vi "caratterizzazione statica.vi"() -> ()   [LabVIEW 2018]
doc: "This example shows how to configure the oscilloscope to perform an edge-triggered waveform acquisition."
uses:
  <vilib>/Analysis/NI_AALBase.lvlib
  <vilib>/Analysis/NI_AALPro.lvlib
  <vilib>/Analysis/1siggen.llb/Ramp Pattern by Samples.vi
  <vilib>/Analysis/baseanly.llb/Mean (DBL).vi
panel:
  out "max  DNL":dbl=0.25455617495711635
  out "max INL":dbl=0.006364783176684707
  out "INL %":dbl[](array[numeric])=[-0.02405619471115613, 0.06846033804956807, 0.054059831701956974, 0.03454117168943075, -0.03038655836860471, -0.0169696576328108, 0.008050584729997558, 0.03499742026747299, 0.02574456923276381, 0.060912347825317355, 0.034353307326495594, 0.07958518493749565, -0.10774409972043486, -0.021201842595099794, 0.020342897229907505, 0.0016005079430486502, -0.009466821478132525, 0.09116154122292272, -0.01932230466677758, -0.09837062153436701, 0.03364044817915108, -0.011195856420213644, -0.039945564937355474, 0.028477623368902888, 0.029414918163196593, -0.028587533779876415, 0.03593350415287439, 0.03881992615814148, -0.02262514986204033, 0.02136618715120852, 0.040058560181039995, -0.01594928109914272, -0.05257185681596037, -0.03030300195705092, 0.026778203505154082, 0.064704262044265, -0.12952305737290118, 0.041345470255055625, 0.10255372792530139, -0.06324005298613465, 0.020945528396060623, -0.10150639984050625, -0.05126306376498192, -0.004301798179200901, -0.05009188774190607, 0.016201328635920543, 0.030310943352047145, 0.008278932638131297, 0.011989906629121232, 0.005500887190787434, 0.05366077708015016, 0.0719716701814557, -0.008277512747636799, 0.013537732291346796, 0.05896730598852085, -0.05698049429107934, -0.004800590826435734, -0.010604611556285334, -0.05143046497149469, -0.0020644348075213583, -0.024163179746751445, 0.2344907926667456, 0.14697455017375938, 0.20964338602529015, 0.16112184156531656, 0.20423462507496437, 0.18626824583724363, 0.1305633884626625, 0.13010680397133367, 0.18381225454299233, 0.10517732744394762, 0.12992217677058013, 0.17510581294016545, 0.19567783989586932, 0.17998590276065332, 0.11545444986578082, 0.25146759119594675, 0.1749255139529328, 0.12922996766805236, 0.2469189617343613, 0.11945547850968391, 0.19403629983585344, 0.23362332282395698, 0.1956925576555358, 0.11779668279024512, 0.194035727637214, 0.12580094899747457, 0.21720642451959113, 0.2745524121266202, 0.06926517425797794, 0.19953514675634204, 0.05343013134212848, 0.2597150989022119, 0.21261490580646905, 0.16132209405759385, 0.26963134998063487, 0.21786887342412437, 0.09562312790087672, 0.19401450852225913, 0.10571657902932799, 0.17270873155994773, 0.19443092071480667, 0.24458001260962836, 0.1318332034488084, 0.1124323203688547, 0.23550485379434946, 0.2375929283663153, 0.2535110917374496, 0.20460950236283787, 0.2178684745299112, 0.05315797518233562, 0.19460595954160134, 0.3034512313480214, 0.2708214826807394, 0.12574594000636555, 0.14251415541887774, 0.05093588968482587, 0.20449728869005027, 0.1926822373705016, 0.26256355176430085, 0.1411123863773901, 0.19777839159011132, 0.21854781672842588, 0.13600196636201495, 0.13105922904496697, 0.4730276164928865, 0.48395264103777597, 0.4650088701146358, 0.4612302792300106, 0.4427108979968476, 0.41475874913826527, 0.4567820701627306, 0.42666815677927117, 0.4296240398582632, 0.4352469807159263, 0.4348952185112967, 0.4715714849603954, 0.4172577117499153, 0.45106984920335297, 0.39335077022924325, 0.4910664907571427, 0.40855424461403156, 0.46358252844017234, 0.42219567309755557, 0.5061272616143334, 0.4030286187935715, 0.37816665716653164, 0.3520374965638744, 0.4195941282659093, 0.40209211632563824, 0.40889141473324186, 0.3932961304753009, 0.4715090833114835, 0.45913995511626593, 0.3216708713005614, 0.5080044439657493, 0.42130251786092243, 0.4439937536246789, 0.5339617639068427, 0.46177970359606074, 0.431955913497639, 0.3944090090598614, 0.4469254776953338, 0.3251812657824317, 0.4115634438057263, 0.3283808796507927, 0.43996795135533545, 0.40160484810391767, 0.4395084238568267, 0.27704803852776005, 0.4648180517939234, 0.3461999727771157, 0.39272858308450964, 0.4152915571086398, 0.3902766058493558, 0.41615611301747524, 0.48392321491798573, 0.41989782766107037, 0.4661658939641799, 0.3360873621634328, 0.4422271917205249, 0.35287120361413, 0.4864596553968769, 0.4345401946028552, 0.4404514982465365, 0.40099996406206806, 0.41323964167756433, 0.46050567969210243, 0.3250850081180961, 0.29173200579040687, 0.3686345298096912, 0.45417118045506755, 0.47477097934735324, 0.522840701958332, 0.4336171377236045, 0.4631331093354117, 0.49692860692656016, 0.38241450435925395, 0.46634222678171283, 0.38182879987710944, 0.42115342284135643, 0.41682029926610015, 0.44335064761131915, 0.3858182444499899, 0.4345787039660407, 0.3827594146281949, 0.4649047016250239, 0.4882343132461272, 0.4304595205210977, 0.38095777001331044, 0.4465832640416022, 0.42807967259696783, 0.328156912962888, 0.5378848734838563, 0.34536408765170046, 0.47744480430399366, 0.388068448334859, 0.4365205750366294, 0.44042771894135235, 0.4016437108627117, 0.4659221314226296, 0.43530939882665803, 0.4350443527613471, 0.4342764357453131, 0.42212656361326234, 0.47592595132213533, 0.3550740108613398, 0.4073838983181634, 0.3838357698978803, 0.4231175566595142, 0.41826335520964203, 0.36262584640439854, 0.38862935896979195, 0.4000631259067917, 0.40127414514936466, 0.5209281999041453, 0.37808863225516304, 0.331143236282089, 0.4095107639232486, 0.4410859342218857, 0.46127773713094705, 0.4116622392192246, 0.39287821593630257, 0.3538630598555873, 0.44490294875246156, 0.3591077799885698, 0.3665597897571065, 0.6364783176684707]
  out "INL":dbl[](array[numeric])=[-0.0002405619471115613, 0.0006846033804956806, 0.0005405983170195698, 0.0003454117168943075, -0.0003038655836860471, -0.000169696576328108, 8.050584729997559e-05, 0.0003499742026747299, 0.0002574456923276381, 0.0006091234782531735, 0.00034353307326495593, 0.0007958518493749565, -0.0010774409972043486, -0.00021201842595099796, 0.00020342897229907507, 1.60050794304865e-05, -9.466821478132525e-05, 0.0009116154122292272, -0.0001932230466677758, -0.0009837062153436702, 0.0003364044817915108, -0.00011195856420213644, -0.00039945564937355477, 0.0002847762336890289, 0.00029414918163196593, -0.00028587533779876416, 0.00035933504152874395, 0.0003881992615814148, -0.00022625149862040328, 0.00021366187151208518, 0.0004005856018104, -0.0001594928109914272, -0.0005257185681596037, -0.0003030300195705092, 0.0002677820350515408, 0.0006470426204426501, -0.0012952305737290119, 0.00041345470255055625, 0.001025537279253014, -0.0006324005298613465, 0.00020945528396060624, -0.0010150639984050625, -0.0005126306376498193, -4.301798179200902e-05, -0.0005009188774190607, 0.00016201328635920544, 0.00030310943352047145, 8.278932638131298e-05, 0.00011989906629121232, 5.5008871907874336e-05, 0.0005366077708015015, 0.000719716701814557, -8.277512747636798e-05, 0.00013537732291346797, 0.0005896730598852085, -0.0005698049429107934, -4.800590826435734e-05, -0.00010604611556285333, -0.0005143046497149469, -2.0644348075213584e-05, -0.00024163179746751446, 0.002344907926667456, 0.001469745501737594, 0.0020964338602529014, 0.0016112184156531655, 0.0020423462507496437, 0.0018626824583724364, 0.001305633884626625, 0.0013010680397133368, 0.0018381225454299232, 0.0010517732744394761, 0.0012992217677058012, 0.0017510581294016543, 0.001956778398958693, 0.0017998590276065332, 0.0011545444986578082, 0.002514675911959467, 0.0017492551395293279, 0.0012922996766805237, 0.002469189617343613, 0.0011945547850968391, 0.0019403629983585342, 0.0023362332282395697, 0.001956925576555358, 0.0011779668279024511, 0.00194035727637214, 0.0012580094899747457, 0.0021720642451959113, 0.0027455241212662016, 0.0006926517425797794, 0.0019953514675634205, 0.0005343013134212847, 0.002597150989022119, 0.0021261490580646906, 0.0016132209405759384, 0.0026963134998063487, 0.0021786887342412436, 0.0009562312790087672, 0.0019401450852225912, 0.00105716579029328, 0.0017270873155994773, 0.0019443092071480667, 0.0024458001260962837, 0.001318332034488084, 0.001124323203688547, 0.0023550485379434946, 0.002375929283663153, 0.0025351109173744964, 0.0020460950236283787, 0.002178684745299112, 0.0005315797518233562, 0.0019460595954160134, 0.0030345123134802136, 0.0027082148268073943, 0.0012574594000636554, 0.0014251415541887773, 0.0005093588968482586, 0.0020449728869005026, 0.001926822373705016, 0.0026256355176430086, 0.001411123863773901, 0.001977783915901113, 0.0021854781672842587, 0.0013600196636201494, 0.0013105922904496697, 0.004730276164928865, 0.00483952641037776, 0.004650088701146358, 0.004612302792300106, 0.004427108979968476, 0.004147587491382653, 0.004567820701627306, 0.004266681567792712, 0.004296240398582632, 0.004352469807159263, 0.004348952185112967, 0.004715714849603954, 0.004172577117499153, 0.00451069849203353, 0.003933507702292433, 0.004910664907571427, 0.004085542446140316, 0.004635825284401723, 0.004221956730975556, 0.005061272616143334, 0.004030286187935715, 0.0037816665716653166, 0.003520374965638744, 0.004195941282659093, 0.004020921163256383, 0.004088914147332419, 0.003932961304753009, 0.004715090833114835, 0.004591399551162659, 0.0032167087130056137, 0.005080044439657493, 0.004213025178609224, 0.004439937536246789, 0.005339617639068427, 0.004617797035960608, 0.00431955913497639, 0.0039440900905986145, 0.004469254776953338, 0.0032518126578243173, 0.004115634438057263, 0.0032838087965079274, 0.0043996795135533544, 0.004016048481039177, 0.004395084238568267, 0.0027704803852776007, 0.004648180517939234, 0.003461999727771157, 0.003927285830845097, 0.004152915571086398, 0.003902766058493558, 0.004161561130174752, 0.0048392321491798574, 0.004198978276610704, 0.004661658939641799, 0.003360873621634328, 0.004422271917205249, 0.0035287120361413, 0.004864596553968769, 0.004345401946028552, 0.004404514982465365, 0.004009999640620681, 0.0041323964167756435, 0.0046050567969210246, 0.003250850081180961, 0.002917320057904069, 0.003686345298096912, 0.004541711804550676, 0.004747709793473533, 0.005228407019583319, 0.004336171377236045, 0.004631331093354117, 0.004969286069265602, 0.0038241450435925394, 0.004663422267817128, 0.003818287998771094, 0.004211534228413564, 0.004168202992661001, 0.004433506476113192, 0.003858182444499899, 0.004345787039660407, 0.003827594146281949, 0.004649047016250239, 0.004882343132461272, 0.004304595205210977, 0.0038095777001331045, 0.004465832640416022, 0.004280796725969678, 0.0032815691296288804, 0.005378848734838563, 0.003453640876517005, 0.004774448043039937, 0.0038806844833485896, 0.004365205750366294, 0.004404277189413524, 0.004016437108627117, 0.004659221314226296, 0.00435309398826658, 0.004350443527613471, 0.004342764357453131, 0.004221265636132623, 0.0047592595132213535, 0.003550740108613398, 0.004073838983181634, 0.0038383576989788034, 0.0042311755665951425, 0.0041826335520964205, 0.0036262584640439854, 0.0038862935896979193, 0.0040006312590679174, 0.0040127414514936465, 0.0052092819990414525, 0.0037808863225516306, 0.00331143236282089, 0.004095107639232486, 0.004410859342218857, 0.00461277737130947, 0.004116622392192246, 0.003928782159363026, 0.003538630598555873, 0.0044490294875246155, 0.003591077799885698, 0.0036655978975710653, 0.006364783176684707]
  out "LSB":dbl=0.078125
  out "DNL":dbl[](array[numeric])=[-0.114720500623298, 0.017856627871037745, 0.02420313841553252, 0.08051038527196397, -0.016636956912384447, -0.031025100529882367, -0.03341407606646953, 0.011473535283039382, -0.043608045454766396, 0.03293321021853899, -0.05608752823764007, 0.23228831297583383, -0.10731239883541548, -0.05151547738300906, 0.02324056271570498, 0.013723488482264656, -0.1247791697493085, 0.13699996890322835, 0.09801991291581089, -0.16369372644476243, 0.05559701770321226, 0.03564963856125587, -0.08484475349976037, -0.0011622455449241897, 0.07192304040941053, -0.08000608703661101, -0.003579163286531184, 0.07619189426502544, -0.054549257896428574, -0.023178542556991033, 0.06944972318742657, 0.045411993888853884, -0.027613380025047717, -0.0707806947731342, -0.04702831258849756, 0.24084187607728608, -0.21187697425866645, -0.07589823951110475, 0.2055842883301807, -0.10439012091392215, 0.15184039101334293, -0.06230173673365016, -0.05823196932636847, 0.05677971105775441, -0.08220358830850501, -0.017495922247996988, 0.02731969328525565, -0.004601607748827519, 0.00804638410353391, -0.05971826346280977, -0.02270550744561888, 0.0995089868320747, -0.027050903848339657, -0.056332671384495825, 0.14377527234670423, -0.06470308029615808, 0.007196985705013504, 0.050624058234859604, -0.061213877403326934, 0.027402443724645308, -0.3207309257927363, 0.10852014069130292, -0.07770935645589816, 0.06016671513036727, -0.05345985155196331, 0.022278310254773715, 0.06907402314448063, 0.0005661647692477345, -0.06659475870885671, 0.09750730960281544, -0.030683613165024326, -0.05602770885028576, -0.025509313425072833, 0.019458002047667834, 0.0800190015896419, -0.16865629524940573, 0.09491217578133729, 0.05666247739325172, -0.14593435264222307, 0.15805471919859998, -0.0924802184444502, -0.04908790850524838, 0.04703414880884225, 0.09659088483296045, -0.09453641561024143, 0.08461112551327687, -0.11334278964742453, -0.071109024632716, 0.25455617495711635, -0.1615347658979715, 0.18117021911362485, -0.2557933597745034, 0.058404239438721105, 0.06360308656860525, -0.13430347734457088, 0.06418547093007305, 0.15158472444882704, -0.12200531197051419, 0.1094894325712346, -0.08307026913796847, -0.026935514552025096, -0.0621848739495789, 0.13980604335941677, 0.024057095019142594, -0.15260994144761356, -0.0025892124692376227, -0.019738522580206565, 0.060637970824518564, -0.016441125487170895, 0.20424101919099372, -0.17539550060548947, -0.13496813703996083, 0.0404608883474296, 0.17989367291622357, -0.020792587111515104, 0.11355704951022431, -0.19041613476647826, 0.014650663636240324, -0.08665282984831109, 0.15059944507976936, -0.07026584646377429, -0.025754087171510065, 0.10235685445434957, 0.006128994273139554, -0.4240408004354202, -0.013547030435663032, 0.023490275944693904, 0.004685452696935144, 0.022964032729122154, 0.03466066458464212, -0.05210891807033704, 0.037341252595489746, -0.003665295017950143, -0.006972446663502297, 0.00043618513374070743, -0.04547857039688239, 0.06734907878099534, -0.04192705044226273, 0.07157165792789613, -0.12116749345459539, 0.10231518521745783, -0.06823507194441447, 0.0513197006248447, -0.10407516976080444, 0.12784231709774474, 0.030828832417529383, 0.03240015914729497, -0.0837702233105233, 0.021702494805936112, -0.008431130025428502, 0.019338152479846826, -0.09698406151686641, 0.015337718962069858, 0.1704616639314736, -0.231053630104833, 0.10751038836998532, -0.028137132347058013, -0.11156033274988317, 0.08950575478536962, 0.03698149972204305, 0.046558161502844086, -0.06512042110798574, 0.15096282277199863, -0.10711390074888527, 0.10314637955211765, -0.13836796891363293, 0.04757024803175795, -0.04700043393360716, 0.2014508778080426, -0.2328348164500426, 0.1470864179808416, -0.05769547678116851, -0.027978087789921346, 0.03101853956151217, -0.03209058888846812, -0.084031206356633, 0.07939148019857498, -0.0573724022158558, 0.16129737943292638, -0.13161338865079414, 0.11080142525192968, -0.16564968021060622, 0.06438013138458701, -0.007330016518164939, 0.04891990238874087, -0.015177200243215339, -0.05860988713802726, 0.1679216327517679, 0.041357722886334616, -0.09535912978391252, -0.10606544680026672, -0.025543750626434304, -0.0596064560376135, 0.11063721965106196, -0.03659980479864089, -0.04190641701302411, 0.14199748718345973, -0.10407037580384895, 0.10479664936170821, -0.04876253247566638, 0.005373073233317882, -0.032897631948071646, 0.07134017992004829, -0.060462969799903024, 0.06425591877892885, -0.10186015587606789, -0.02892871841016813, 0.07164074297903653, 0.06138217062965623, -0.08137561259508175, 0.022944453391346542, 0.12390422194625898, -0.26006267104600056, 0.2387257744318731, -0.1637800886488435, 0.110826681401727, -0.06008063711019531, -0.004844858441856559, 0.04809217001751449, -0.07970524149429821, 0.037959788419004784, 0.00032865712098555376, 0.0009522170998820911, 0.015065841443743011, -0.06671124075900252, 0.14985640617138643, -0.06486426044646124, 0.029199679241150987, -0.0487094155844261, 0.00601920979784154, 0.06899051091850197, -0.032244355581087805, -0.014177871001879793, -0.0015016638607903588, -0.1483710278959279, 0.17712106388473786, 0.05821229100661185, -0.09717573427503794, -0.03915321117030999, -0.025037835607236048, 0.06152321741053583, 0.02329218887082334, 0.048378793540086916, -0.11288946223212407, 0.10638600926722575, -0.009240492112985521, -0.3346989746100917]
  in  "Tab Control":T1(tab)=enum."CONFRONTO IDEALE E REALE"
  out "confonto":waveform(dbl)[](graph)=[{"t0"=timestamp(0 s since 1904-01-01), "dt"=0.004968040310037549, "Y"=array[248 elements]}, {"t0"=timestamp(0 s since 1904-01-01), "dt"=0.004968040310037549, "Y"=array[248 elements]}]
  out "caratteristica statica":cluster{dbl[], dbl[]}(graph)
  out "confronto_rette":waveform(dbl)[](graph)=[{"t0"=timestamp(0 s since 1904-01-01), "dt"=0.004968040310037549, "Y"=array[248 elements]}, {"t0"=timestamp(0 s since 1904-01-01), "dt"=0.004968040310037549, "Y"=array[248 elements]}]
  out "errore di guadagno":dbl=-0.03778591631762984
  out "errore di offset":dbl=-0.0867022391606219
  out "indice di fine":i32[](array[numeric])=[14456, 16723, 18456, 21505, 23709, 26413, 29108, 31158, 33625, 36266, 38593, 40967, 43393, 45899, 48260, 50985, 53393, 55786, 58394, 61024, 63323, 65806, 68077, 70558, 73011, 75148, 77531, 80438, 83009, 85630, 87816, 89884, 92915, 95362, 97565, 100055, 102725, 105116, 107615, 109890, 112715, 114748, 117411, 119927, 122388, 124611, 127009, 129720, 132220, 134440, 137028, 139689, 142241, 144479, 147120, 149302, 151791, 154288, 156401, 158906, 161200, 161840, 163991, 166805, 168779, 171154, 173963, 176799, 178820, 181316, 183821, 186240, 188493, 190897, 193657, 195968, 198386, 200815, 203476, 205711, 208132, 210856, 213165, 215518, 218224, 220352, 223130, 225234, 227710, 230461, 232827, 235213, 237556, 240076, 242612, 245335, 247884, 249961, 252449, 255007, 257485, 260368, 262124, 264905, 267237, 269451, 272112, 274533, 276764, 279531, 281913, 284275, 286601, 289404, 291680, 294136, 296699, 299289, 301701, 304247, 306668, 309055, 311414, 313809, 316282, 318363, 320936, 323678, 325761, 328350, 330813, 333525, 335679, 338193, 340678, 343038, 345661, 347935, 350198, 352729, 355358, 357454, 360316, 362728, 364986, 367659, 369996, 372569, 374882, 377422, 379681, 382098, 384776, 386954, 389560, 392053, 394753, 397195, 399599, 402323, 404450, 406924, 409239, 411743, 414037, 416556, 419129, 421576, 424003, 426770, 428845, 431509, 433963, 436150, 438972, 441177, 443554, 446420, 448927, 451100, 453904, 456074, 458409, 460997, 463092, 465352, 467869, 470586, 472925, 474843, 477222, 479813, 482368, 484728, 487359, 489650, 492193, 494678, 497046, 499683, 502458, 504340, 506860, 509357, 512055, 514236, 517014, 519521, 521613, 524185, 526630, 529244, 531831, 533968, 536546, 538865, 541776, 543881, 546333, 548925, 551386, 554006, 556481, 558698, 561061, 563619, 566039, 568728, 571076, 573756, 576131, 578465, 580633, 583168, 585776, 588224, 590660, 593170, 596000, 598189, 600599, 602951, 605989, 607859, 610435, 612874, 615271, 616036]
  out "min value":dbl=-9.765625
  out "max value":dbl=9.6875
  out "numeri di bit eq":dbl=8.0
  out "Mediane\n delle transizioni":dbl[](array[numeric])=[-9.711754383605852, -9.628450693829347, -9.563160577563249, -9.482094657483247, -9.402734254100897, -9.318823887343532, -9.240546693360889, -9.173558042212518, -9.086142774343122, -8.999841370558375, -8.933272006793093, -8.856738023732786, -8.773977577473183, -8.697079406873614, -8.61836308611707, -8.537818585337915, -8.45963081566549, -8.380008308714919, -8.305852108986114, -8.226776401564537, -8.147385386819485, -8.063110453034081, -7.992749471086037, -7.918102548036758, -7.8318115234375, -7.758912816811036, -7.6826498035363455, -7.605517818132168, -7.524312187775492, -7.438687001182383, -7.370851277101277, -7.2942079835606854, -7.208347315436241, -7.13753003203417, -7.0553024933288855, -6.977843198016734, -6.8980551010244735, -6.818803543613707, -6.747076277068295, -6.668486563773111, -6.580164210074413, -6.518291975881262, -6.435745709714951, -6.351214960390006, -6.269655577447711, -6.205167767732963, -6.117637662639405, -6.041772527100271, -5.962948616315941, -5.889512310606061, -5.8112699370793095, -5.726219533922463, -5.643830796497081, -5.5773093250070165, -5.495097268790165, -5.415857919254658, -5.332570329087049, -5.255821078431373, -5.181534090909091, -5.102868210306407, -5.019800275482094, -4.966740262681159, -4.88468137254902, -4.793696609717031, -4.726530136702569, -4.655189479638009, -4.563558467741935, -4.4846746333897345, -4.408865770210057, -4.332170514319111, -4.262139545223577, -4.178438065781533, -4.108913745387454, -4.017409500339904, -3.9443576860401954, -3.869053002894356, -3.7851304188096986, -3.715886377613776, -3.634807378266033, -3.5635558684054534, -3.4804461994868507, -3.3906963005215123, -3.317048373287671, -3.237247816139767, -3.1634347960444993, -3.0865077554744524, -3.007653617083091, -2.9284452296819787, -2.8515897212543555, -2.770127118644068, -2.697134067357513, -2.619495476366322, -2.5488352479941647, -2.4585282397782398, -2.393628003003003, -2.301866460637606, -2.2168218510230178, -2.1481579830053668, -2.0776494060876023, -1.9934338521400778, -1.9142027099784638, -1.8290969681129117, -1.7661413257277734, -1.6785218598195697, -1.6078115638106651, -1.5233654289667897, -1.4471704345273046, -1.3757402368758003, -1.2886949315654406, -1.2061106687898089, -1.133898384673178, -1.0544518288084463, -0.9794178598342125, -0.8953067200986436, -0.8196829432079816, -0.7485795454545454, -0.6641673657718121, -0.5897458217270195, -0.5060948581560284, -0.42627245508982037, -0.3540540072102052, -0.2712673611111111, -0.1934148264984227, -0.12478081162324649, -0.04931294326241135, 0.01962819778541428, 0.09187700029095142, 0.17405523255813954, 0.2466143428747307, 0.3293353873239437, 0.409167921686747, 0.49038392343120324, 0.5589087511325883, 0.6450269033087054, 0.7237224430113978, 0.7991752001847859, 0.8738205946239479, 0.9510988609813084, 1.0331075174825175, 1.1025232812927965, 1.193955866727383, 1.2645524222381124, 1.3461640869071287, 1.4225535558146314, 1.4956722474905897, 1.5865265376984128, 1.6529498922413792, 1.7277175350436393, 1.8039060323209808, 1.8990197224820704, 1.9655420676582094, 2.050463237788331, 2.117670203790239, 2.208102154046997, 2.289998811033608, 2.359254360880755, 2.4440541714947854, 2.518349723090031, 2.591874651907547, 2.674368564993565, 2.745297585626053, 2.8192620103229222, 2.902835700330628, 2.9789595170454546, 3.05321250721709, 3.12722255770263, 3.219967995759948, 3.2934160656461584, 3.3678232758620688, 3.4548046980774436, 3.516169717082328, 3.6074509410563174, 3.685823516889015, 3.7612781268264173, 3.839204616637434, 3.9180570610096006, 3.9940007831145583, 4.08481835399449, 4.160177342062635, 4.234902426160337, 4.321937769010043, 4.384071021928592, 4.468474860982391, 4.561700386789646, 4.618910424305919, 4.692457507082153, 4.771928792361485, 4.861704465541491, 4.941709844559585, 5.014073149951314, 5.095332829925651, 5.174446749654218, 5.246905979918658, 5.329749888259833, 5.40919678147939, 5.48263143776824, 5.5652769866135, 5.638174862448418, 5.716356402528668, 5.799642559689062, 5.8805637406947895, 5.946947782920275, 6.02677319876647, 6.109089921807124, 6.182066077760892, 6.266436002764128, 6.347696603822314, 6.420555134041477, 6.502976190476191, 6.584933483935743, 6.654728084415584, 6.731294775197629, 6.808154273297924, 6.8862526633522725, 6.971515326778484, 7.045321377840909, 7.131132309217047, 7.201062620556627, 7.2745652887139105, 7.362013813467282, 7.432948435972629, 7.525845390309556, 7.591424546713674, 7.675149150049036, 7.750260569046226, 7.825229960578187, 7.901683293937708, 7.986540421195652, 8.056343454879329, 8.140026325805634, 8.221902105484052, 8.29412798272079, 8.376196997162673, 8.455096316680779, 8.523932963588136, 8.610032306846302, 8.686717692828147, 8.766010641985579, 8.851975565582105, 8.915021315658452, 8.999592391304347, 9.078675560570764, 9.160938219052001, 9.22901774003148, 9.310064409632314, 9.389618288590604, 9.47034502423724, 9.521046789617486]
  out "indice di inizio":i32[](array[numeric])=[9808, 13336, 15452, 17476, 20478, 22818, 25237, 27723, 30390, 32917, 35060, 37554, 40037, 42291, 44997, 47493, 49997, 52401, 54577, 57189, 59833, 62197, 64532, 66967, 69811, 72031, 74477, 76776, 79606, 82247, 84449, 87025, 89190, 91616, 94567, 96828, 99211, 101906, 104013, 106699, 109221, 111514, 113973, 116645, 119089, 121016, 123781, 126030, 128751, 131140, 133611, 136181, 138644, 140916, 143541, 146082, 148494, 150616, 153101, 155316, 157933, 160184, 162716, 164932, 167572, 170049, 172413, 175026, 177249, 179605, 181853, 184583, 187138, 189426, 191816, 194586, 197025, 199189, 201792, 204024, 206573, 209322, 211705, 214316, 216606, 218982, 221409, 224102, 226275, 228986, 231476, 233859, 236185, 238633, 240947, 243798, 246320, 248843, 251102, 253722, 256092, 258455, 260853, 263464, 265568, 268367, 270409, 272971, 275595, 277961, 280582, 282949, 285274, 287782, 290377, 292541, 295209, 297494, 300291, 302577, 304865, 307579, 309829, 312312, 314449, 315744, 317499, 320023, 322512, 324800, 327493, 330051, 332368, 335080, 337344, 339791, 341978, 344511, 347195, 349078, 352064, 354657, 356795, 359297, 361798, 364635, 366516, 368788, 371293, 374215, 376252, 379150, 380924, 384273, 386406, 388556, 391301, 393674, 396008, 398438, 400888, 403146, 405912, 408223, 410573, 412830, 416063, 418179, 420378, 423077, 425116, 428082, 430440, 432728, 434981, 437948, 440202, 442790, 445223, 447782, 450419, 452517, 455172, 457636, 459274, 461822, 464151, 467031, 469644, 471762, 473994, 476198, 478434, 481372, 483817, 486155, 488682, 491043, 493645, 496081, 498428, 500991, 503293, 505904, 508107, 510980, 513142, 515567, 518442, 520699, 522780, 525196, 527689, 530448, 533088, 535345, 537740, 540252, 542523, 545242, 547294, 550291, 552510, 555639, 557643, 559814, 562443, 565048, 567264, 569815, 572557, 574819, 577461, 579625, 581629, 584587, 586965, 589564, 592066, 594172, 597149, 599517, 601643, 604047, 606573, 609149, 611764, 614206]
  out "RAMPA":dbl[](graph)
  in  "length":i32=1400000
  in  "Vertical Coupling (0: A1M)":u16(ring)=2 items=["A1M", "A50", "D1M", "D50", "Ground"]
  in  "Probe Attenuation (1X)":dbl=1.0
  in  "Vertical Range (1 V)":dbl=2.0
  in  "Trigger Level (0.0 V)":dbl
  in  "Timebase (0.0005 s)":dbl=0.2
  in  "Source (1: Channel 1)":u16(ring)=1 items=["Channel 1"=1, "Channel 2"=2, "Channel 3"=3, "Channel 4"=4]
  in  "VISA resource name":refnum<visa-resource-name>="USB0::0xF4EC::0xEE38::SDSMMEBX3R2562::INSTR"
  # "PARAMETRI DELL'ADC"
  # "CARATTERIZZAZIONE STATICA"
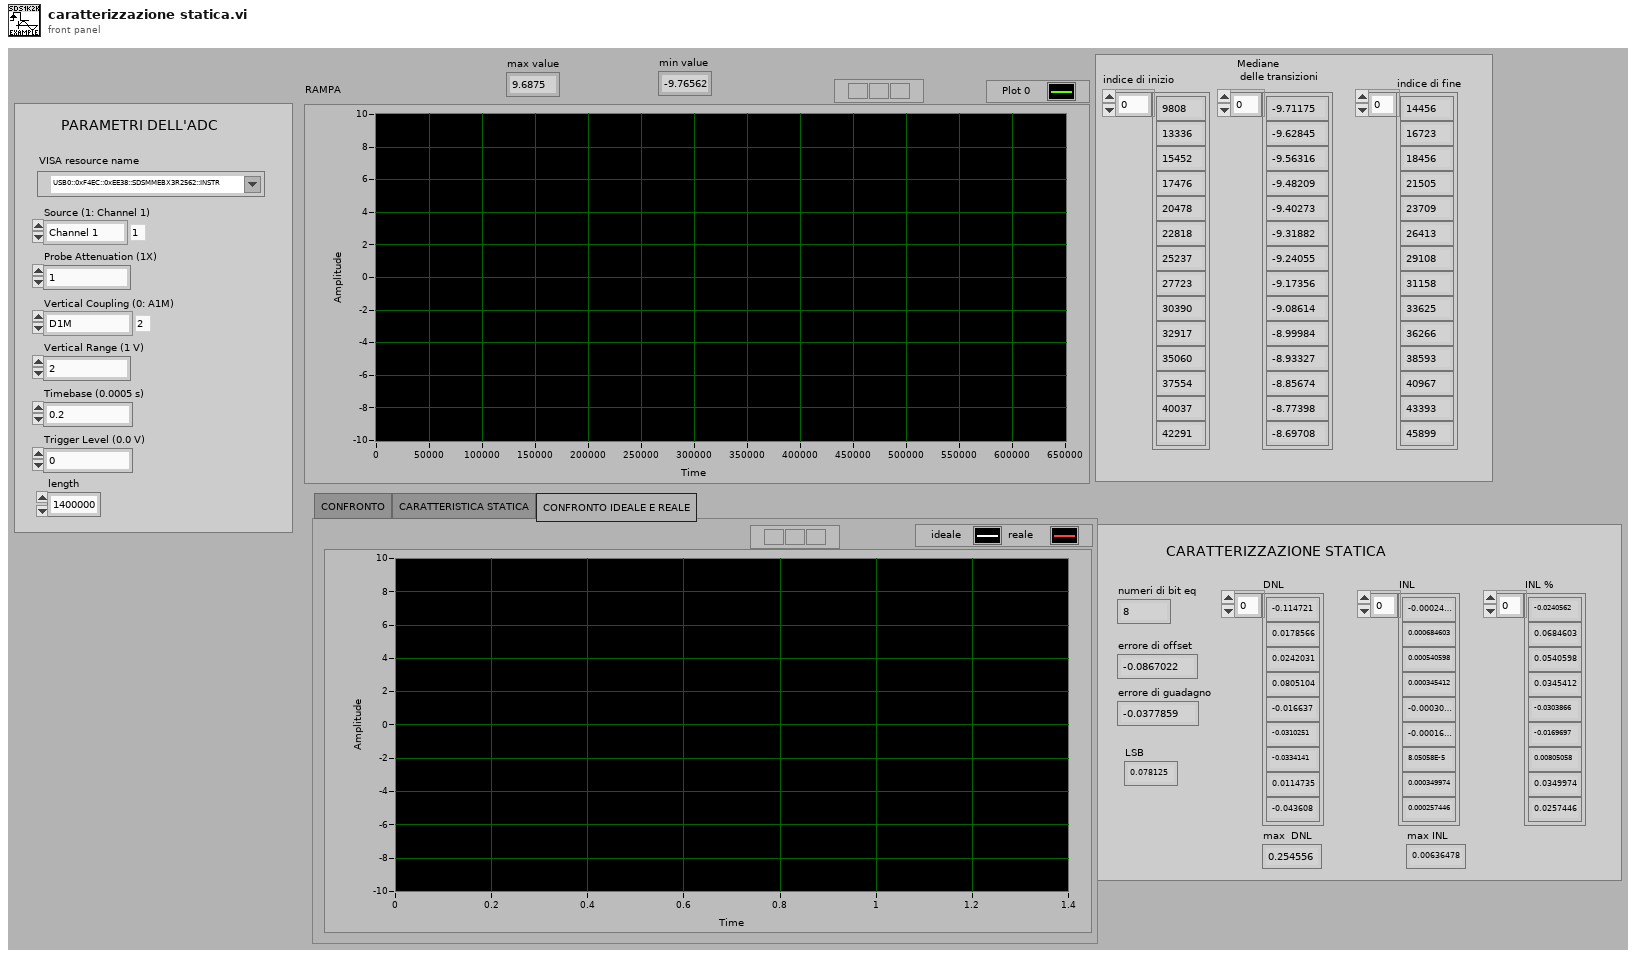
[diagram p1: front panel]
types:
  T1 = enum32{"CONFRONTO", "CARATTERISTICA STATICA", "CONFRONTO IDEALE E REALE"}
  T2 = cluster{"Best Linear Fit":dbl[], "Ramp Pattern":dbl[]}
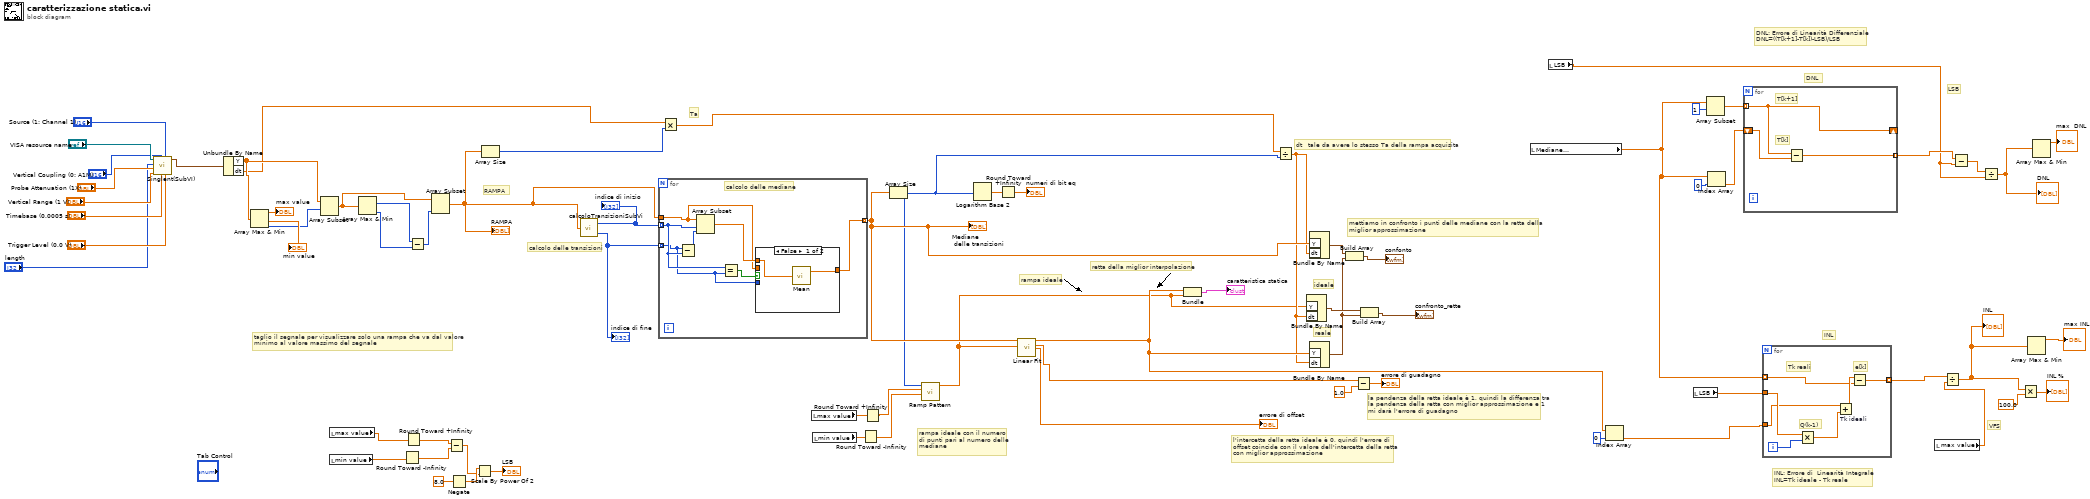
[diagram p0: block diagram]
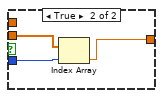
[diagram p2: hidden frame]
diagram:
  # "reale"
  # "ideale"
  # "INL: Errore di  Linearità Integrale\nINL=Tk ideale - Tk reale"
  # "VFS"
  # "INL"
  # "DNL: Errore di Linearità Differenziale\nDNL=((T[k+1]-T[k])-LSB)/LSB"
  # "LSB"
  # "DNL"
  # "rampa ideale con il numero\ndi punti pari al numero delle\nmediane"
  # "mettiamo in confronto i punti delle mediane con la retta della\nmiglior approssimazione"
  # "la pendenza della retta ideale è 1, quindi la differenza tra\nla pendenza della retta con miglior approssimazione e 1 \nmi darà l'errore di guadagno"
  # "l'intercetta della retta ideale è 0, quindi l'errore di \noffset coincide con il valore dell'intercetta della retta\ncon miglior approssimazione"
  # "rampa ideale"
  # "retta della miglior interpolazione"
  # "RAMPA"
  # "taglio il segnale per visualizzare solo una rampa che va dal valore\nminimo al valore massimo del segnale"
  # "calcolo delle transizioni"
  # "dt   tale da avere lo stesso Ta della rampa acquisita"
  # "Ta"
  n1 = call "Singlent(SubVI).vi"("Trigger Level (0.0 V)"="Trigger Level (0.0 V)", "Source (1: Channel 1)"="Source (1: Channel 1)", "Timebase (0.0005 s)"="Timebase (0.0005 s)", "Vertical Coupling (0: A1M)"="Vertical Coupling (0: A1M)", "Vertical Range (1 V)"="Vertical Range (1 V)", "Probe Attenuation (1X)"="Probe Attenuation (1X)", "length"="length", "VISA Refnum in"="VISA resource name") -> ("Waveform Graph"=w5:waveform(dbl))  [unwired: 3 in]
  n2 = Unbundle By Name(w5) -> ("Y"=w60:dbl[], "dt"=w47:dbl)
  n3 = Array Max & Min(array=w60) -> (max value=→"max value":dbl, min value=→"min value":dbl, min index (indices)=w55:i32)  [unwired: 1 out]
  n4 = Array Subset(array=w60, index=w55) -> (w51:dbl[])  [unwired: 1 in]
  n5 = local read "max value"() -> (w13:dbl)
  n6 = local read "min value"() -> (w12:dbl)
  n7 = Array Max & Min(array=w51) -> (max index (indices)=w52:i32, min index (indices)=w53:i32)  [unwired: 2 out]
  n8 = Round Toward -Infinity(1:w12) -> (0:w14:dbl)
  n9 = Round Toward +Infinity(x=w13) -> (ceil(x): smallest int >= x=w15:dbl)
  n10 = Subtract(x=w52, y=w53) -> (x-y=w54:i32)
  n11 = Array Subset(array=w51, length=w54) -> (w48:dbl[])  [unwired: 1 in]
  "RAMPA" <- w48
  n12 = Subtract(x=w15, y=w14) -> (x-y=w30:dbl)
  n13 = Negate(x=8.0) -> (-x=w31:dbl)
  n14 = Scale By Power Of 2(n=w31, x=w30) -> (x*2^n=→"LSB":dbl)
  n15 = Array Size(array=w48) -> (size(s)=w7:i32)
  n16 = call "calcoloTransizioniSubVi.vi"("Array"=w48) -> ("indice di inizio"=w57:i32[], "indice di fine"=w56:i32[])
  "indice di inizio" <- w57
  "indice di fine" <- w56
  n17 = for {
    tunnel: w48 -> [w74]
    tunnel: w57 -> [w73] mode=indexing
    tunnel: w56 -> [w72] mode=indexing
    tunnel: [w75] -> w45 mode=indexing
    # "calcolo delle mediane"
    n18 = Subtract(x=w72, y=w73) -> (x-y=w78:i32)
    n19 = Array Subset(array=w74, index=w73, length=w78) -> (w76:dbl[])
    n20 = Equal?(x=w73, y=w72) -> (x = y?=w77:bool)
    n21 = case shown="False" w77 {
      tunnel: w76 -> [w80 _]
      tunnel: [w79 w83] -> w75
      tunnel: w74 -> [_ w82]
      tunnel: w72 -> [_ w81]
      frame False {
        n22 = call-poly <vilib>:"Mean.vi"("X"=w80) -> ("mean"=w79:dbl)  [unwired: 1 out]
      }
      frame True {
        n23 = Index Array(array=w82, index=w81) -> (element=w83:dbl)
      }
    }
  }
  "Mediane\n delle transizioni" <- w45
  n24 = Multiply(x=w47, y=w7) -> (x*y=w46:dbl)
  n25 = local read "max value"() -> (w43:dbl)
  n26 = local read "min value"() -> (w42:dbl)
  n27 = Round Toward -Infinity(1:w42) -> (0:w16:dbl)
  n28 = Round Toward +Infinity(x=w43) -> (ceil(x): smallest int >= x=w17:dbl)
  n29 = Array Size(array=w45) -> (size(s)=w44:i32)
  n30 = call-poly <vilib>:"Ramp Pattern.vi"("start"=w16, "end"=w17, "samples"=w44) -> ("Ramp Pattern"=w6:dbl[])  [unwired: 7 in, 1 out]
  n31 = Logarithm Base 2(1:w44) -> (0:w63:dbl)
  n32 = Round Toward +Infinity(x=w63) -> (ceil(x): smallest int >= x=→"numeri di bit eq":dbl)
  n33 = call <vilib>:"Linear Fit.vi"("Y"=w45, "X"=w6) -> ("Best Linear Fit"=w19:dbl[], "slope"=w40:dbl, "intercept"=→"errore di offset":dbl)  [unwired: 9 in, 2 out]
  n34 = Bundle("Best Linear Fit"=w19, "Ramp Pattern"=w6) -> (→"caratteristica statica":T2)  [unwired: 1 in]
  n35 = Divide(x=w46, y=w44) -> (x/y=w11:dbl)
  n36 = Bundle By Name("Y"=w6, "dt"=w11) -> (w10:waveform(dbl))  [unwired: 1 in]
  n37 = Bundle By Name("Y"=w45, "dt"=w11) -> (w50:waveform(dbl))  [unwired: 1 in]
  n38 = Bundle By Name("Y"=w19, "dt"=w11) -> (w9:waveform(dbl))  [unwired: 1 in]
  n39 = Build Array(w50, w9) -> (→"confonto":waveform(dbl)[])
  n40 = Subtract(x=w40, y=1.0) -> (x-y=→"errore di guadagno":dbl)
  n41 = Build Array(w10, w9) -> (→"confronto_rette":waveform(dbl)[])
  n42 = local read "Mediane\n delle transizioni"() -> (w21:dbl[])
  n43 = local read "LSB"() -> (w27:dbl)
  n44 = Index Array(array=w19, index=0) -> (element=w18:dbl)
  n45 = local read "LSB"() -> (w22:dbl)
  n46 = Array Subset(array=w21, index=1) -> (w35:dbl[])  [unwired: 1 in]
  n47 = Index Array(array=w21, index=0) -> (element=w33:dbl)
  n48 = for {
    tunnel: w35 -> [w86] mode=indexing
    shift-right: [w86] -> _
    shift-left: w33 -> [w85]
    tunnel: [w84] -> w32 mode=indexing
    # "T[k]"
    # "T[k+1]"
    n49 = Subtract(x=w86, y=w85) -> (x-y=w84:dbl)
  }
  n50 = for {
    tunnel: w18 -> [w90]
    tunnel: w21 -> [w87] mode=indexing
    tunnel: w22 -> [w92]
    tunnel: [w89] -> w23 mode=indexing
    i -> [w93]
    # "Tk reali"
    # "e[k]"
    # "Q(k-1)"
    n51 = Multiply(x=w92, y=w93) -> (x*y=w91:dbl)
    n52 = Add "Tk ideali"(x=w90, y=w91) -> (x+y=w88:dbl)
    n53 = Subtract(x=w88, y=w87) -> (x-y=w89:dbl)
  }
  n54 = local read "max value"() -> (w25:dbl)
  n55 = Divide(x=w23, y=w25) -> (x/y=w3:dbl[])
  "INL" <- w3
  n56 = Subtract(x=w32, y=w27) -> (x-y=w34:dbl[])
  n57 = Divide(x=w34, y=w27) -> (x/y=w4:dbl[])
  "DNL" <- w4
  n58 = Multiply(x=w3, y=100.0) -> (x*y=→"INL %":dbl[])
  n59 = Array Max & Min(array=w3) -> (max value=→"max INL":dbl)  [unwired: 3 out]
  n60 = Array Max & Min(array=w4) -> (max value=→"max  DNL":dbl)  [unwired: 3 out]
